vi "Open Subview VI Reference.vi"(8 "error in (no error)":errorcluster, 11 "Subview String":string) -> (0 "error out":errorcluster, 3 "Subview VI Reference":refnum<vi>)   [LabVIEW 2024]
doc: "Opens the subview VI reference."
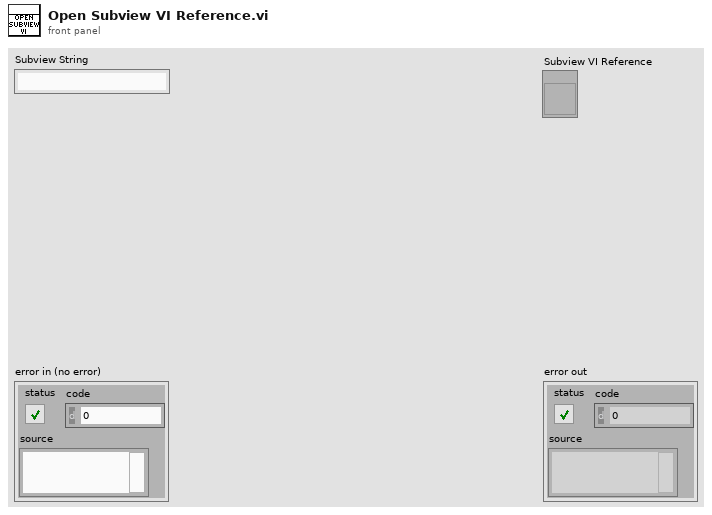
[diagram p1: front panel]
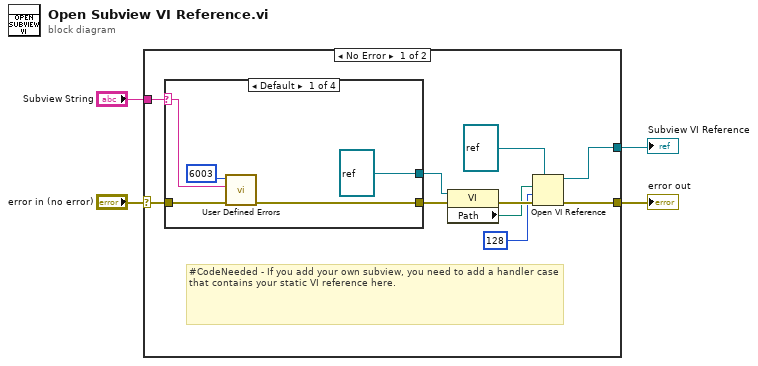
[diagram p0: block diagram]
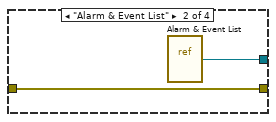
[diagram p2: hidden frame]
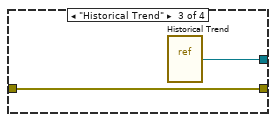
[diagram p3: hidden frame]
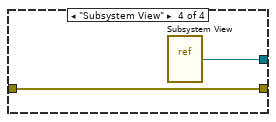
[diagram p4: hidden frame]
diagram:
  n1 = case shown="No Error" "error in (no error)" {
    selector: "error in (no error)" -> [w13 w26]
    tunnel: "Subview String" -> [w14 _]
    tunnel: [w8 w26] -> w2
    tunnel: [w7 _] -> w1
    frame No Error {
      # "#CodeNeeded - If you add your own subview, you need to add a handler case that contains your static VI reference here."
      n2 = case shown="Default" w14 {
        selector: w14 -> [w17 _ _ _]
        tunnel: w13 -> [w19 w21 w23 w25]
        tunnel: [w18 w21 w23 w25] -> w12
        tunnel: [refnum<vi> refnum w20 w22 w24] -> w6
        frame Default {
          n3 = call "User Defined Errors.vi"("error in (no error)"=w19, "Parameter 1"=w17, "Error Code (0)"=6003 ("error code (0)")) -> ("error out"=w18:errorcluster)  [unwired: 8 in]
        }
        frame "Alarm & Event List" {
          n4 = vi-ref "Alarm & Event List.vi"() -> (w20:refnum<vi>)
        }
        frame "Historical Trend" {
          n5 = vi-ref "Historical Trend.vi"() -> (w22:refnum<vi>)
        }
        frame "Subsystem View" {
          n6 = vi-ref "Subsystem View.vi"() -> (w24:refnum<vi>)
        }
      }
      n7 = property class="VI"(reference=w6, error in=w12) -> (error out=w11:errorcluster, "Path"=w10:path)  [unwired: 1 out]
      n8 = Open VI Reference(type specifier VI Refnum (for type only)=refnum<vi> refnum, vi path=w10, options=128, error in (no error)=w11) -> (vi reference=w7:refnum<vi>, error out=w8:errorcluster)  [unwired: 2 in]
    }
    frame Error {
    }
  }
  "error out" <- w2
  "Subview VI Reference" <- w1
